vi "Unregister Sessions.vi"(8 "error in":errorcluster, 11 "request data":T2) -> (0 "error out":errorcluster, 3 "response data":T1)   [LabVIEW 2020, in "MeasurementLink Session Management.lvlib"]
uses:
  MeasurementLink Session Management.lvlib
  MeasurementLink gRPC Utilities/gRPC Client Pool Helpers/Action.ctl
  MeasurementLink gRPC Utilities/MeasurementLink gRPC Utilities.lvlib
  MeasurementLink Session Management Client/MeasurementLink Session Management Client.lvlib
  MeasurementLink Session Management Client/RPC Messages/ni_measurementlink_sessionmanagement_v1_ChannelMapping.ctl
  MeasurementLink Session Management Client/RPC Messages/nidevice_grpc_Session.ctl
  MeasurementLink Session Management Client/RPC Messages/ni_measurementlink_sessionmanagement_v1_SessionInformation.ctl
  MeasurementLink Session Management Client/RPC Messages/ni_measurementlink_sessionmanagement_v1_UnregisterSessionsRequest.ctl
  MeasurementLink Session Management Client/RPC Messages/ni_measurementlink_sessionmanagement_v1_UnregisterSessionsResponse.ctl
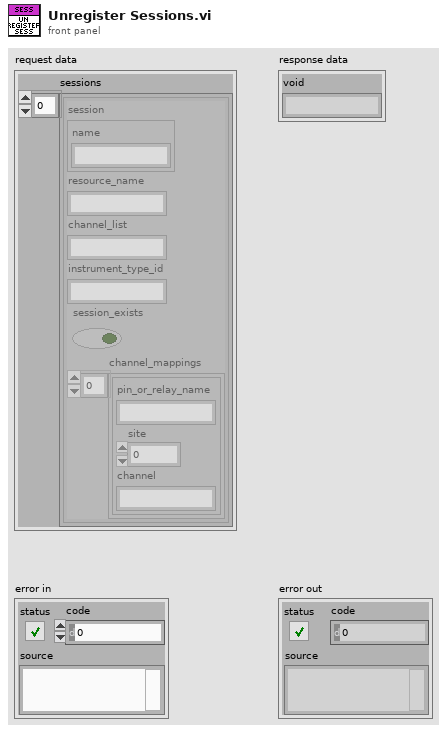
[diagram p1: front panel]
types:
  T1 = typedef "MeasurementLink Session Management Client.lvlib/ni_measurementlink_sessionmanagement_v1_UnregisterSessionsResponse.ctl" = cluster{"void":string}
  T2 = typedef "MeasurementLink Session Management Client.lvlib/ni_measurementlink_sessionmanagement_v1_UnregisterSessionsRequest.ctl" = cluster{"sessions":T3[]}
  T3 = typedef "MeasurementLink Session Management Client.lvlib/ni_measurementlink_sessionmanagement_v1_SessionInformation.ctl" = cluster{"session":T4, "resource_name":string, "channel_list":string, "instrument_type_id":string, "session_exists":bool, "channel_mappings":T5[]}
  T4 = typedef "MeasurementLink Session Management Client.lvlib/nidevice_grpc_Session.ctl" = cluster{"name":string}
  T5 = typedef "MeasurementLink Session Management Client.lvlib/ni_measurementlink_sessionmanagement_v1_ChannelMapping.ctl" = cluster{"pin_or_relay_name":string, "site":i32, "channel":string}
  T6 = typedef "MeasurementLink gRPC Utilities.lvlib/Action.ctl" = enum16{"Get Client", "Recreate Client"}
  T7 = typedef "grpc-lvsupport-release.lvlib/grpcId.ctl" = u64
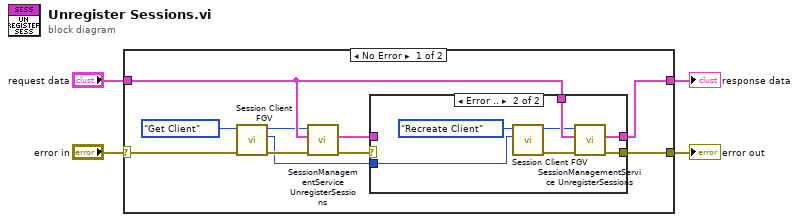
[diagram p0: block diagram]
diagram:
  n1 = case shown="No Error" "error in" {
    selector: "error in" -> [w14 w24]
    tunnel: [w11 w24] -> w3
    tunnel: "request data" -> [w7 _]
    tunnel: [w9 _] -> w1
    frame No Error {
      n2 = call "Session Client FGV.vi"("error in"=w14, "action"=Action."Get Client") -> ("error out"=w13:errorcluster, "unique id out"=w5:u64, "grpc client id"=w6:T7)  [unwired: 7 in]
      n3 = call "SessionManagementService UnregisterSessions.vi"("error in"=w13, "Request Data"=w7, "gRPC ID"=w6) -> ("error out"=w12:errorcluster, "Response Data"=w8:T1)  [unwired: 6 in, 1 out]
      n4 = case shown="Error .." w12 {
        selector: w12 -> [w16 _]
        tunnel: [w16 w22] -> w11
        tunnel: [w15 w21] -> w9
        tunnel: w8 -> [w15 _]
        tunnel: w7 -> [_ w20]
        tunnel: w5 -> [_ w17]
        frame No Error {
        }
        frame Error {
          n5 = call "Session Client FGV.vi"("unique id in"=w17, "action"=Action."Recreate Client") -> ("error out"=w23:errorcluster, "grpc client id"=w19:T7)  [unwired: 7 in, 1 out]
          n6 = call "SessionManagementService UnregisterSessions.vi"("error in"=w23, "Request Data"=w20, "gRPC ID"=w19) -> ("error out"=w22:errorcluster, "Response Data"=w21:T1)  [unwired: 6 in, 1 out]
        }
      }
    }
    frame Error {
    }
  }
  "error out" <- w3
  "response data" <- w1
